vi "UnsimulateAll.vi"(0 "error in":errorcluster, 5 "Telnet":refnum<k24>) -> (4 "error out":errorcluster, 6 "KclCommand":string, 10 "Succeed":bool, 15 "ErrorText":string)   [LabVIEW 2014, in "UnderAutomation.Fanuc.lvlib"]
uses:
  UnderAutomation.Fanuc.lvlib
  C:/Users/fg/Documents/Fanuc.vi/LabVIEW_2024/UnderAutomation.Fanuc/lib/UnderAutomation.Fanuc.dll
  LabVIEW_2024/UnderAutomation.Fanuc/lib/UnderAutomation.Fanuc.dll
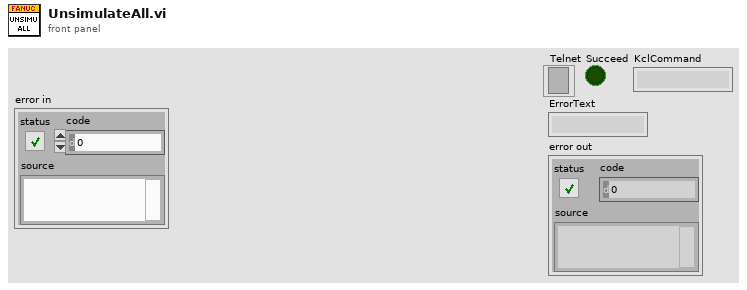
[diagram p1: front panel]
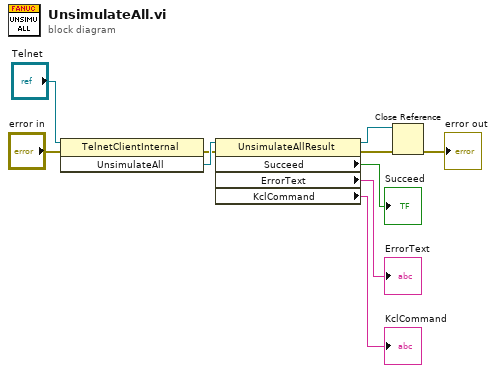
[diagram p0: block diagram]
diagram:
  n1 = invoke class="TelnetClientInternal" method="UnsimulateAll"(reference="Telnet", error in="error in") -> (error out=w6:errorcluster, "UnsimulateAll"=w9:refnum<k24>)  [unwired: 1 in, 1 out]
  n2 = property class="UnsimulateAllResult"(reference=w9, error in=w6) -> (reference out=w2:refnum<k24>, error out=w3:errorcluster, "Succeed"=→"Succeed":bool, "ErrorText"=→"ErrorText":string, "KclCommand"=→"KclCommand":string)
  n3 = Close Reference(reference=w2, error in (no error)=w3) -> (error out=→"error out":errorcluster)
